vi "Final Project.vi"() -> ()   [LabVIEW 2015]
uses:
  <vilib>/NXT/Block Support/NXT_OutputPort.ctl
  <vilib>/NXT/Block Support/NXT_InputPort.ctl
  <vilib>/NXT/Subs/ColorSensorColors.ctl
  <vilib>/NXT/Dual Mode Library/Waits/Wait_Loud.vi
  <vilib>/NXT/Dual Mode Library/Sensors/EV3_Color_Color.vi
  <vilib>/NXT/NXTIO Xnodes/NXTIONodeSubVIs/NXTMoveMotors.vi
  <vilib>/NXT/Dual Mode Library/Waits/Wait_Num.vi
  <vilib>/NXT/Dual Mode Library/Sensors/Reset_Timer.vi
  <vilib>/NXT/Dual Mode Library/Sensors/Read_Timer.vi
  <vilib>/NXT/Dual Mode Library/Sensors/Light_On.vi
  <vilib>/NXT/NXTIO Xnodes/NXTIONodeSubVIs/NXTStopMotors.vi
  <vilib>/NXT/Dual Mode Library/Sound/Tone.vi
  <vilib>/NXT/Dual Mode Library/Waits/Wait_Rotation.vi
  <vilib>/NXT/Dual Mode Library/Sensors/Touch_Pressed.vi
  <vilib>/NXT/Dual Mode Library/Sound/PlayRedPianoFile.vi
  <vilib>/NXT/NXTIO Xnodes/AddressXNode/NXTIOAddress.xnode
  <vilib>/NXT/NXTIO Xnodes/NXTIOXNode/NXTIO.xnode
  <vilib>/NXT/Subs/LVHSConnector.ctl
  <vilib>/NXT/LegoClasses/BrickReference/BrickReference.lvclass
panel:
  out "Scaled Value 6":i16
  out "Scaled Value 5":i16
  out "Scaled Value 4":i16
  out "Scaled Value 3":i16
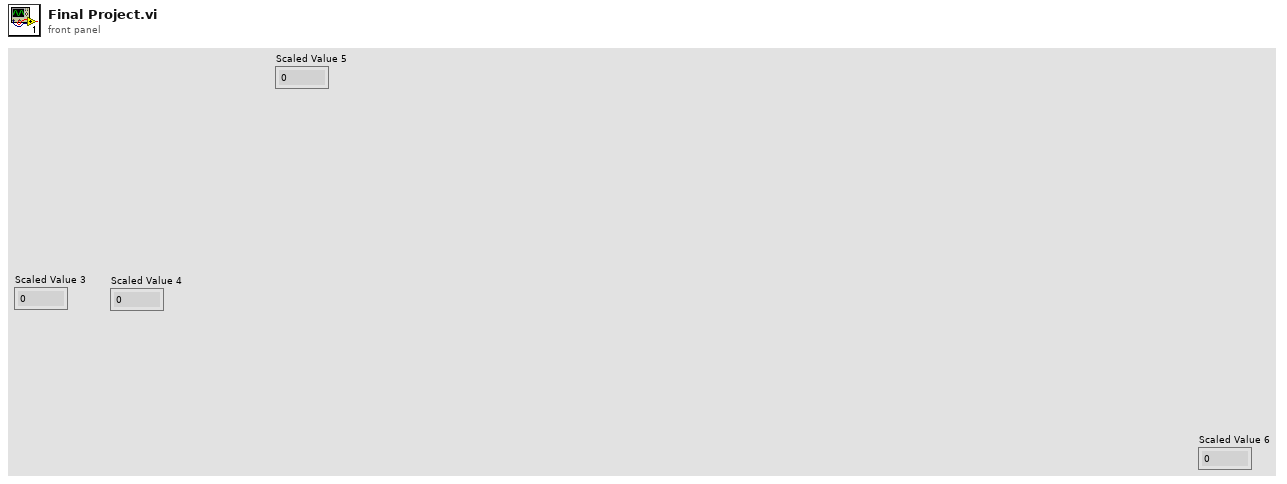
[diagram p1: front panel]
types:
  T1 = typedef "NXT_InputPort.ctl" = u32
  T2 = typedef "LVHSConnector.ctl" = refnum<class "BrickReference.lvclass">
  T3 = typedef "ColorSensorColors.ctl" = enum16{"No Color", "Black", "Blue", "Green", "Yellow", "Red", "White", "Brown"}
  T4 = typedef "NXT_OutputPort.ctl" = u8
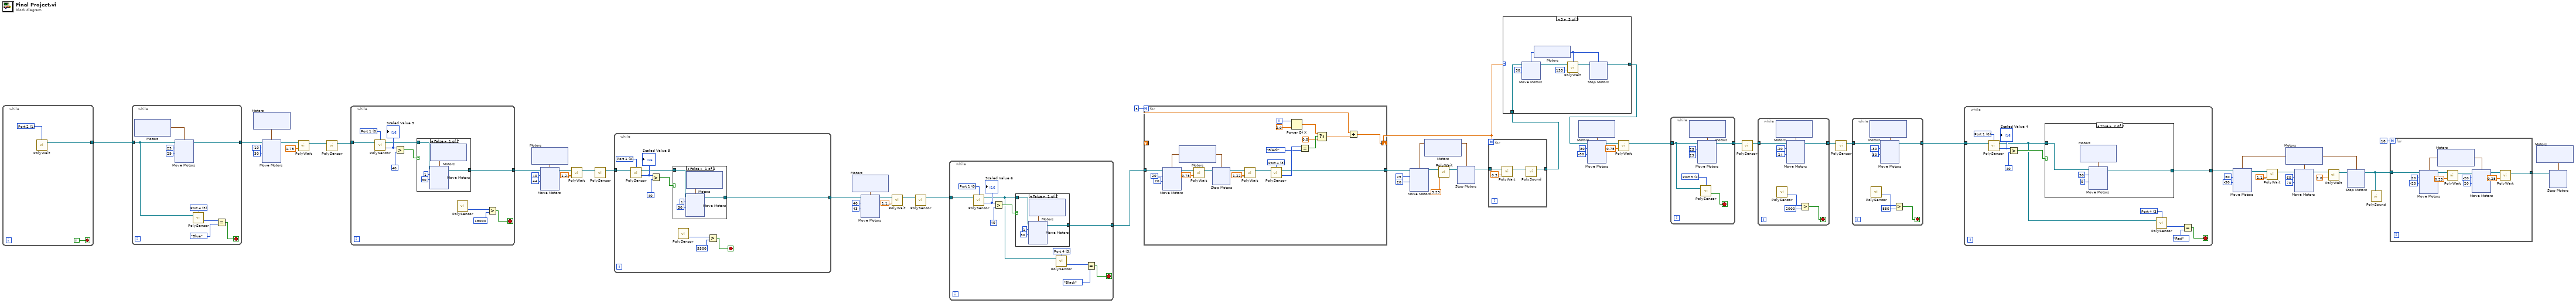
[diagram p0: block diagram]
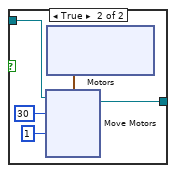
[diagram p2: hidden frame]
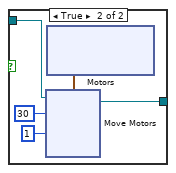
[diagram p3: hidden frame]
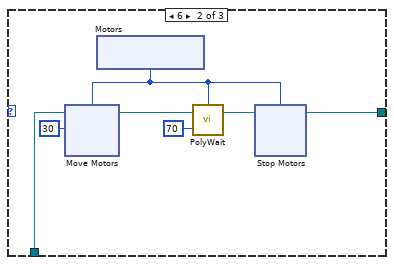
[diagram p5: hidden frame]
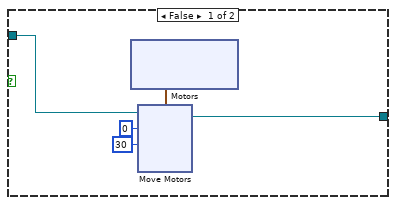
[diagram p6: hidden frame]
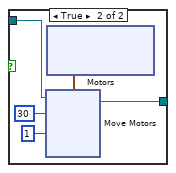
[diagram p7: hidden frame]
diagram:
  n1 = while {
    tunnel: [w67] -> w58
    stop <- TRUE stop-if-true
    w68 = T1 1 items=["Port 1", "Port 2", "Port 3", "Port 4"] ("Port (Port 2)")
    n2 = call-poly <vilib>:"PolyWait.vi"("Port (Port 2)"=w68) -> ("NXT/EV3"=w67:T2)  [unwired: 3 in]
  }
  n3 = while {
    tunnel: w58 -> [w74]
    tunnel: [w73] -> w53
    stop <- w70 stop-if-true
    w71 = T1 3 items=["Port 1", "Port 2", "Port 3", "Port 4"] ("Port (Port 1)")
    n4 = xnode "Motors"() -> ("Motor"=w77:cluster{"Port":T4, "Port":T4})
    n5 = xnode "Move Motors"("Power/Speed 2"=i8 29, "Power/Speed 1"=i8 25 ("Power/Speed 2"), "Motors"=w77, "NXT/EV3"=w74) -> ("NXT/EV3"=w73:T2)
    n6 = call-poly <vilib>:"PolySensor.vi"("NXT/EV3"=w74, "Port (Port 1)"=w71) -> ("Detected Color"=w76:T3)  [unwired: 1 in, 1 out]
    n7 = Equal?(x=w76, y=ColorSensorColors."Blue") -> (x = y?=w70:bool)
  }
  n8 = xnode "Motors"() -> ("Motor"=w56:cluster{"Port":T4, "Port":T4})
  n9 = xnode "Move Motors"("Power/Speed 2"=i8 30, "Power/Speed 1"=i8 -10, "Motors"=w56, "NXT/EV3"=w53) -> ("NXT/EV3"=w51:T2)
  n10 = call-poly <vilib>:"PolyWait.vi"("Time (1 sec)"=sgl 1.75, "NXT/EV3"=w51) -> ("NXT/EV3"=w42:T2)  [unwired: 2 in]
  n11 = call-poly <vilib>:"PolySensor.vi"("NXT/EV3"=w42) -> ("NXT/EV3"=w41:T2)  [unwired: 3 in]
  n12 = while {
    tunnel: [w90] -> w43
    tunnel: w41 -> [w89]
    stop <- w91 stop-if-true
    w93 = T1 0 items=["Port 1", "Port 2", "Port 3", "Port 4"] ("Port (Port 3)")
    n13 = call-poly <vilib>:"PolySensor.vi"("NXT/EV3"=w89, "Port (Port 3)"=w93) -> ("Scaled Value"=w96:i16, "NXT/EV3"=w88:T2)  [unwired: 1 in]
    "Scaled Value 3" <- w96
    n14 = Greater?(x=w96, y=i16 40 ("Scaled Value")) -> (0:w94:bool)
    n15 = case shown="False" w94 {
      tunnel: w88 -> [w98 w111]
      tunnel: [w97 w112] -> w90
      frame False {
        n16 = xnode "Motors"() -> ("Motor"=w101:cluster{"Port":T4, "Port":T4})
        n17 = xnode "Move Motors"("Power/Speed 2"=i8 30, "Power/Speed 1"=i8 1, "Motors"=w101, "NXT/EV3"=w98) -> ("NXT/EV3"=w97:T2)
      }
      frame True {
        n18 = xnode "Motors"() -> ("Motor"=w115:cluster{"Port":T4, "Port":T4})
        n19 = xnode "Move Motors"("Power/Speed 2"=i8 1, "Power/Speed 1"=i8 30, "Motors"=w115, "NXT/EV3"=w111) -> ("NXT/EV3"=w112:T2)
      }
    }
    n20 = call-poly <vilib>:"PolySensor.vi"() -> ("Value (msec)"=w92:u32)  [unwired: 3 in, 1 out]
    n21 = Greater?(x=w92, y=u32 18000) -> (0:w91:bool)
  }
  n22 = xnode "Motors"() -> ("Motor"=w40:cluster{"Port":T4, "Port":T4})
  n23 = xnode "Move Motors"("Power/Speed 2"=i8 44, "Power/Speed 1"=i8 40, "Motors"=w40, "NXT/EV3"=w43) -> ("NXT/EV3"=w37:T2)
  n24 = call-poly <vilib>:"PolyWait.vi"("Time (1 sec)"=sgl 1.3, "NXT/EV3"=w37) -> ("NXT/EV3"=w35:T2)  [unwired: 2 in]
  n25 = call-poly <vilib>:"PolySensor.vi"("NXT/EV3"=w35) -> ("NXT/EV3"=w34:T2)  [unwired: 3 in]
  n26 = while {
    tunnel: [w128] -> w26
    tunnel: w34 -> [w127]
    stop <- w129 stop-if-true
    w131 = T1 0 items=["Port 1", "Port 2", "Port 3", "Port 4"] ("Port (Port 3)")
    n27 = call-poly <vilib>:"PolySensor.vi"("NXT/EV3"=w127, "Port (Port 3)"=w131) -> ("Scaled Value"=w134:i16, "NXT/EV3"=w126:T2)  [unwired: 1 in]
    "Scaled Value 5" <- w134
    n28 = Greater?(x=w134, y=i16 40 ("Scaled Value")) -> (0:w132:bool)
    n29 = case shown="False" w132 {
      tunnel: w126 -> [w136 w149]
      tunnel: [w135 w150] -> w128
      frame False {
        n30 = xnode "Motors"() -> ("Motor"=w139:cluster{"Port":T4, "Port":T4})
        n31 = xnode "Move Motors"("Power/Speed 2"=i8 30, "Power/Speed 1"=i8 1, "Motors"=w139, "NXT/EV3"=w136) -> ("NXT/EV3"=w135:T2)
      }
      frame True {
        n32 = xnode "Motors"() -> ("Motor"=w153:cluster{"Port":T4, "Port":T4})
        n33 = xnode "Move Motors"("Power/Speed 2"=i8 1, "Power/Speed 1"=i8 30, "Motors"=w153, "NXT/EV3"=w149) -> ("NXT/EV3"=w150:T2)
      }
    }
    n34 = call-poly <vilib>:"PolySensor.vi"() -> ("Value (msec)"=w130:u32)  [unwired: 3 in, 1 out]
    n35 = Greater?(x=w130, y=u32 5500) -> (0:w129:bool)
  }
  n36 = xnode "Motors"() -> ("Motor"=w32:cluster{"Port":T4, "Port":T4})
  n37 = xnode "Move Motors"("Power/Speed 2"=i8 43, "Power/Speed 1"=i8 40, "Motors"=w32, "NXT/EV3"=w26) -> ("NXT/EV3"=w29:T2)
  n38 = call-poly <vilib>:"PolyWait.vi"("Time (1 sec)"=sgl 1.1, "NXT/EV3"=w29) -> ("NXT/EV3"=w27:T2)  [unwired: 2 in]
  n39 = call-poly <vilib>:"PolySensor.vi"("NXT/EV3"=w27) -> ("NXT/EV3"=w25:T2)  [unwired: 3 in]
  n40 = while {
    tunnel: [w168] -> w33
    tunnel: w25 -> [w167]
    stop <- w169 stop-if-true
    w164 = T1 3 items=["Port 1", "Port 2", "Port 3", "Port 4"] ("Port (Port 1)")
    w170 = T1 0 items=["Port 1", "Port 2", "Port 3", "Port 4"] ("Port (Port 3)")
    n41 = call-poly <vilib>:"PolySensor.vi"("NXT/EV3"=w167, "Port (Port 3)"=w170) -> ("Scaled Value"=w173:i16, "NXT/EV3"=w163:T2)  [unwired: 1 in]
    "Scaled Value 6" <- w173
    n42 = Greater?(x=w173, y=i16 40 ("Scaled Value")) -> (0:w171:bool)
    n43 = case shown="False" w171 {
      tunnel: w163 -> [w175 w188]
      tunnel: [w174 w189] -> w168
      frame False {
        n44 = xnode "Motors"() -> ("Motor"=w178:cluster{"Port":T4, "Port":T4})
        n45 = xnode "Move Motors"("Power/Speed 2"=i8 30, "Power/Speed 1"=i8 1, "Motors"=w178, "NXT/EV3"=w175) -> ("NXT/EV3"=w174:T2)
      }
      frame True {
        n46 = xnode "Motors"() -> ("Motor"=w192:cluster{"Port":T4, "Port":T4})
        n47 = xnode "Move Motors"("Power/Speed 2"=i8 1, "Power/Speed 1"=i8 30, "Motors"=w192, "NXT/EV3"=w188) -> ("NXT/EV3"=w189:T2)
      }
    }
    n48 = call-poly <vilib>:"PolySensor.vi"("NXT/EV3"=w163, "Port (Port 1)"=w164) -> ("Detected Color"=w166:T3)  [unwired: 1 in, 1 out]
    n49 = Equal?(x=w166, y=ColorSensorColors."Black") -> (x = y?=w169:bool)
  }
  n50 = for {
    N: 3 -> [_]
    tunnel: w33 -> [w223]
    shift-right: [w208] -> w44
    shift-left: _ -> [w209]
    tunnel: [w207] -> w63
    i -> [w211]
    w206 = T1 3 items=["Port 1", "Port 2", "Port 3", "Port 4"] ("Port (Port 1)")
    n51 = xnode "Motors"() -> ("Motor"=w218:cluster{"Port":T4, "Port":T4})
    n52 = xnode "Move Motors"("Power/Speed 2"=i8 20, "Power/Speed 1"=i8 20, "Motors"=w218, "NXT/EV3"=w223) -> ("NXT/EV3"=w221:T2)
    n53 = call-poly <vilib>:"PolyWait.vi"("Time (1 sec)"=sgl 0.75, "NXT/EV3"=w221) -> ("NXT/EV3"=w219:T2)  [unwired: 2 in]
    n54 = xnode "Stop Motors"("Motors"=w218, "NXT/EV3"=w219) -> ("NXT/EV3"=w204:T2)
    n55 = call-poly <vilib>:"PolyWait.vi"("Time (1 sec)"=sgl 1.22, "NXT/EV3"=w204) -> ("NXT/EV3"=w203:T2)  [unwired: 2 in]
    n56 = call-poly <vilib>:"PolySensor.vi"("NXT/EV3"=w203, "Port (Port 1)"=w206) -> ("Detected Color"=w217:T3, "NXT/EV3"=w207:T2)  [unwired: 1 in]
    n57 = Power Of X(1:2.0 ("x"), 2:w211) -> (0:w212:dbl)
    n58 = Equal?(x=w217, y=ColorSensorColors."Black") -> (x = y?=w215:bool)
    n59 = Select(t=w212, s=w215, f=0.0) -> (s? t:f=w210:dbl)
    n60 = Add(x=w209, y=w210) -> (x+y=w208:dbl)
  }
  n61 = xnode "Motors"() -> ("Motor"=w57:cluster{"Port":T4, "Port":T4})
  n62 = xnode "Move Motors"("Power/Speed 2"=i8 20, "Power/Speed 1"=i8 25 ("Power/Speed 2"), "Motors"=w57, "NXT/EV3"=w63) -> ("NXT/EV3"=w61:T2)
  n63 = call-poly <vilib>:"PolyWait.vi"("Time (1 sec)"=sgl 3.25, "NXT/EV3"=w61) -> ("NXT/EV3"=w60:T2)  [unwired: 2 in]
  n64 = xnode "Stop Motors"("Motors"=w57, "NXT/EV3"=w60) -> ("NXT/EV3"=w59:T2)
  n65 = for {
    N: w44 -> [_]
    tunnel: [w240] -> w23
    tunnel: w59 -> [w238]
    n66 = call-poly <vilib>:"PolyWait.vi"("Time (1 sec)"=sgl 0.3, "NXT/EV3"=w238) -> ("NXT/EV3"=w241:T2)  [unwired: 2 in]
    n67 = call-poly <vilib>:"PolySound.vi"("NXT/EV3"=w241) -> ("NXT/EV3"=w240:T2)  [unwired: 3 in]
  }
  n68 = case shown="5" w44 {
    tunnel: w23 -> [w242 w246 w266]
    tunnel: [w242 w244 w264] -> w22
    frame 7, Default {
    }
    frame 6 {
      n69 = xnode "Motors"() -> ("Motor"=w243:T4)
      n70 = xnode "Move Motors"("Power/Speed 1"=i8 30, "Motors"=w243, "NXT/EV3"=w246) -> ("NXT/EV3"=w248:T2)
      n71 = call-poly <vilib>:"PolyWait.vi"("Position Change (180)"=70, "NXT/EV3"=w248, "Port (Port A)"=w243) -> ("NXT/EV3"=w245:T2)  [unwired: 1 in]
      n72 = xnode "Stop Motors"("Motors"=w243, "NXT/EV3"=w245) -> ("NXT/EV3"=w244:T2)
    }
    frame 5 {
      n73 = xnode "Motors"() -> ("Motor"=w263:T4)
      n74 = xnode "Move Motors"("Power/Speed 1"=i8 30, "Motors"=w263, "NXT/EV3"=w266) -> ("NXT/EV3"=w268:T2)
      n75 = call-poly <vilib>:"PolyWait.vi"("Position Change (180)"=155, "NXT/EV3"=w268, "Port (Port A)"=w263) -> ("NXT/EV3"=w265:T2)  [unwired: 1 in]
      n76 = xnode "Stop Motors"("Motors"=w263, "NXT/EV3"=w265) -> ("NXT/EV3"=w264:T2)
    }
  }
  n77 = xnode "Motors"() -> ("Motor"=w49:cluster{"Port":T4, "Port":T4})
  n78 = xnode "Move Motors"("Power/Speed 2"=i8 -30, "Power/Speed 1"=i8 30, "Motors"=w49, "NXT/EV3"=w22) -> ("NXT/EV3"=w46:T2)
  n79 = call-poly <vilib>:"PolyWait.vi"("Time (1 sec)"=sgl 0.75, "NXT/EV3"=w46) -> ("NXT/EV3"=w24:T2)  [unwired: 2 in]
  n80 = while {
    tunnel: w24 -> [w284]
    tunnel: [w283] -> w21
    stop <- w285 stop-if-true
    w286 = T1 2 items=["Port 1", "Port 2", "Port 3", "Port 4"] ("Port (Port 1)")
    n81 = xnode "Motors"() -> ("Motor"=w289:cluster{"Port":T4, "Port":T4})
    n82 = xnode "Move Motors"("Power/Speed 2"=i8 29, "Power/Speed 1"=i8 25, "Motors"=w289, "NXT/EV3"=w284) -> ("NXT/EV3"=w283:T2)
    n83 = call-poly <vilib>:"PolySensor.vi"("NXT/EV3"=w284, "Port (Port 1)"=w286) -> ("Yes / No"=w285:bool)  [unwired: 1 in, 1 out]
  }
  n84 = call-poly <vilib>:"PolySensor.vi"("NXT/EV3"=w21) -> ("NXT/EV3"=w20:T2)  [unwired: 3 in]
  n85 = while {
    tunnel: w20 -> [w303]
    tunnel: [w302] -> w19
    stop <- w299 stop-if-true
    n86 = xnode "Motors"() -> ("Motor"=w306:cluster{"Port":T4, "Port":T4})
    n87 = call-poly <vilib>:"PolySensor.vi"() -> ("Value (msec)"=w301:u32)  [unwired: 3 in, 1 out]
    n88 = xnode "Move Motors"("Power/Speed 2"=i8 -24, "Power/Speed 1"=i8 -20, "Motors"=w306, "NXT/EV3"=w303) -> ("NXT/EV3"=w302:T2)
    n89 = Greater?(x=w301, y=u32 2000) -> (0:w299:bool)
  }
  n90 = call-poly <vilib>:"PolySensor.vi"("NXT/EV3"=w19) -> ("NXT/EV3"=w18:T2)  [unwired: 3 in]
  n91 = while {
    tunnel: w18 -> [w320]
    tunnel: [w319] -> w17
    stop <- w316 stop-if-true
    n92 = xnode "Motors"() -> ("Motor"=w323:cluster{"Port":T4, "Port":T4})
    n93 = call-poly <vilib>:"PolySensor.vi"() -> ("Value (msec)"=w318:u32)  [unwired: 3 in, 1 out]
    n94 = xnode "Move Motors"("Power/Speed 2"=i8 30, "Power/Speed 1"=i8 -30, "Motors"=w323, "NXT/EV3"=w320) -> ("NXT/EV3"=w319:T2)
    n95 = Greater?(x=w318, y=u32 850) -> (0:w316:bool)
  }
  n96 = while {
    tunnel: [w335] -> w64
    tunnel: w17 -> [w334]
    stop <- w336 stop-if-true
    w339 = T1 3 items=["Port 1", "Port 2", "Port 3", "Port 4"] ("Port (Port 3)")
    w340 = T1 0 items=["Port 1", "Port 2", "Port 3", "Port 4"] ("Port (Port 3)")
    n97 = call-poly <vilib>:"PolySensor.vi"("NXT/EV3"=w334, "Port (Port 3)"=w340) -> ("Scaled Value"=w343:i16, "NXT/EV3"=w333:T2)  [unwired: 1 in]
    "Scaled Value 4" <- w343
    n98 = Greater?(x=w343, y=i16 40 ("Scaled Value")) -> (0:w341:bool)
    n99 = case shown="True" w341 {
      tunnel: w333 -> [w345 w359]
      tunnel: [w344 w358] -> w335
      frame False {
        n100 = xnode "Motors"() -> ("Motor"=w348:cluster{"Port":T4, "Port":T4})
        n101 = xnode "Move Motors"("Power/Speed 2"=i8 30, "Power/Speed 1"=i8 0, "Motors"=w348, "NXT/EV3"=w345) -> ("NXT/EV3"=w344:T2)
      }
      frame True {
        n102 = xnode "Motors"() -> ("Motor"=w362:cluster{"Port":T4, "Port":T4})
        n103 = xnode "Move Motors"("Power/Speed 2"=i8 0, "Power/Speed 1"=i8 30, "Motors"=w362, "NXT/EV3"=w359) -> ("NXT/EV3"=w358:T2)
      }
    }
    n104 = call-poly <vilib>:"PolySensor.vi"("NXT/EV3"=w333, "Port (Port 1)"=w339) -> ("Detected Color"=w338:T3)  [unwired: 1 in, 1 out]
    n105 = Equal?(x=w338, y=ColorSensorColors."Red" ("Detected Color")) -> (x = y?=w336:bool)
  }
  n106 = xnode "Motors"() -> ("Motor"=w1:cluster{"Port":T4, "Port":T4})
  n107 = xnode "Move Motors"("Power/Speed 2"=i8 -30, "Power/Speed 1"=i8 30, "Motors"=w1, "NXT/EV3"=w64) -> ("NXT/EV3"=w14:T2)
  n108 = call-poly <vilib>:"PolyWait.vi"("Time (1 sec)"=sgl 1.1, "NXT/EV3"=w14) -> ("NXT/EV3"=w11:T2)  [unwired: 2 in]
  n109 = xnode "Move Motors"("Power/Speed 2"=i8 70, "Power/Speed 1"=i8 60, "Motors"=w1, "NXT/EV3"=w11) -> ("NXT/EV3"=w9:T2)
  n110 = call-poly <vilib>:"PolyWait.vi"("Time (1 sec)"=sgl 2.0, "NXT/EV3"=w9) -> ("NXT/EV3"=w2:T2)  [unwired: 2 in]
  n111 = xnode "Stop Motors"("Motors"=w1, "NXT/EV3"=w2) -> ("NXT/EV3"=w3:T2)
  n112 = call-poly <vilib>:"PolySound.vi"("NXT/EV3"=w3) -> ()  [unwired: 3 in, 1 out]
  n113 = for {
    N: 18 -> [_]
    tunnel: w3 -> [w372]
    tunnel: [w373] -> w6
    n114 = xnode "Motors"() -> ("Motor"=w381:cluster{"Port":T4, "Port":T4})
    n115 = xnode "Move Motors"("Power/Speed 2"=i8 -20, "Power/Speed 1"=i8 20, "Motors"=w381, "NXT/EV3"=w372) -> ("NXT/EV3"=w376:T2)
    n116 = call-poly <vilib>:"PolyWait.vi"("Time (1 sec)"=sgl 0.25, "NXT/EV3"=w376) -> ("NXT/EV3"=w375:T2)  [unwired: 2 in]
    n117 = xnode "Move Motors"("Power/Speed 2"=i8 20, "Power/Speed 1"=i8 -20, "Motors"=w381, "NXT/EV3"=w375) -> ("NXT/EV3"=w374:T2)
    n118 = call-poly <vilib>:"PolyWait.vi"("Time (1 sec)"=sgl 0.25, "NXT/EV3"=w374) -> ("NXT/EV3"=w373:T2)  [unwired: 2 in]
  }
  n119 = xnode "Motors"() -> ("Motor"=w5:cluster{"Port":T4, "Port":T4})
  n120 = xnode "Stop Motors"("Motors"=w5, "NXT/EV3"=w6) -> ()  [unwired: 1 out]
